vi "FGV_REWORK_DIAGNOSTICS_message_history_buffer.vi"(7 "options":T3, 8 "error_in":errorcluster, 11 "input":variant) -> (0 "error_out":errorcluster, 3 "message_history":T1[](array[typedef]))   [LabVIEW 2019]
uses:
  FGV_REWORK_DIAGNOSTICS_message_history_buffer.ctl
  REWORK_DIAGNOSTICS_message_history_buffer_all_info.ctl
  _misc/DIAGNOSTICS_message_type.ctl
  <userlib>/_OpenG.lib/array/array.llb/Filter 1D Array with Scalar (Variant)__ogtk.vi
  <vilib>/addons/database/_DB Variant To Data/Database Variant To Data.xnode
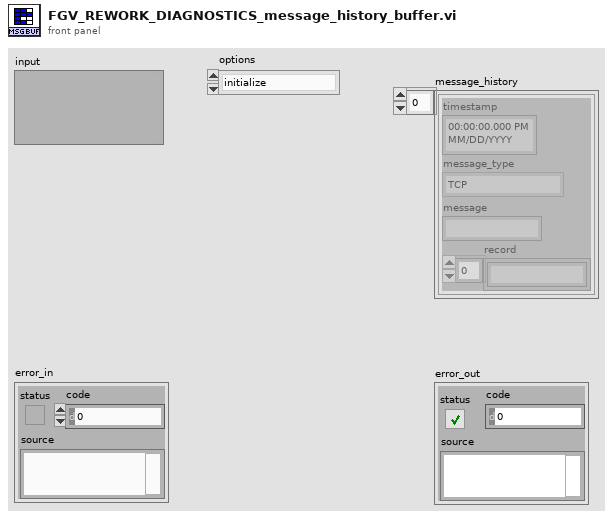
[diagram p1: front panel]
types:
  T1 = typedef "REWORK_DIAGNOSTICS_message_history_buffer_all_info.ctl" = cluster{"timestamp":timestamp, "message_type":T2, "message":string, "record":string[]}
  T2 = typedef "DIAGNOSTICS_message_type.ctl" = enum16{"TCP", "SQL"}
  T3 = typedef "FGV_REWORK_DIAGNOSTICS_message_history_buffer.ctl" = enum16{"initialize", "add_TCP_PLC_to_PC", "add_TCP_PC_to_PLC", "add_SQL_PC_to_DB", "add_SQL_transaction", "add_SQL_DB_to_PC", "get_all", "clear_all", "save_log"}
  T4 = enum16{"open", "replace", "create", "open or create", "replace or create", "replace or create with confirmation"}
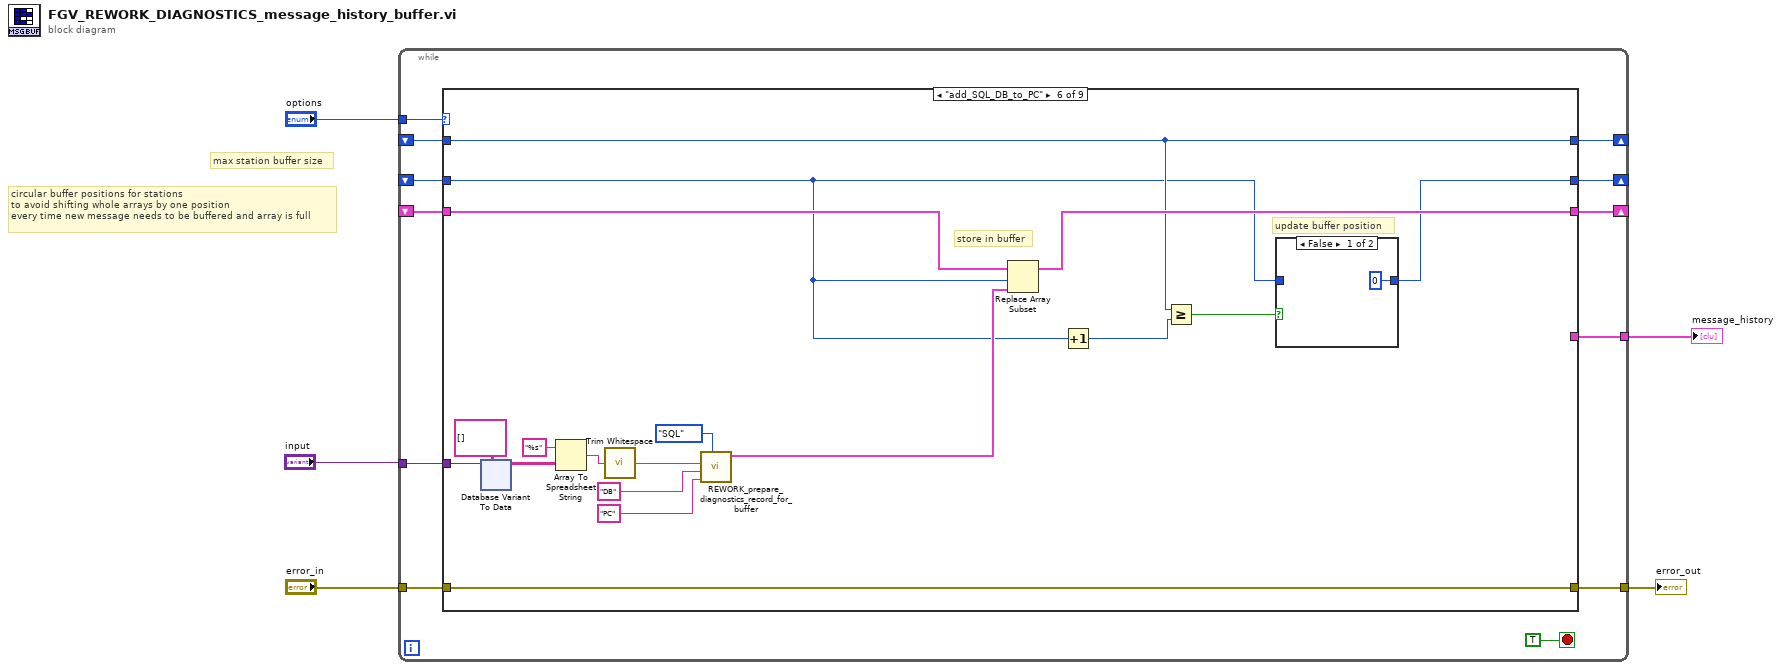
[diagram p0: block diagram]
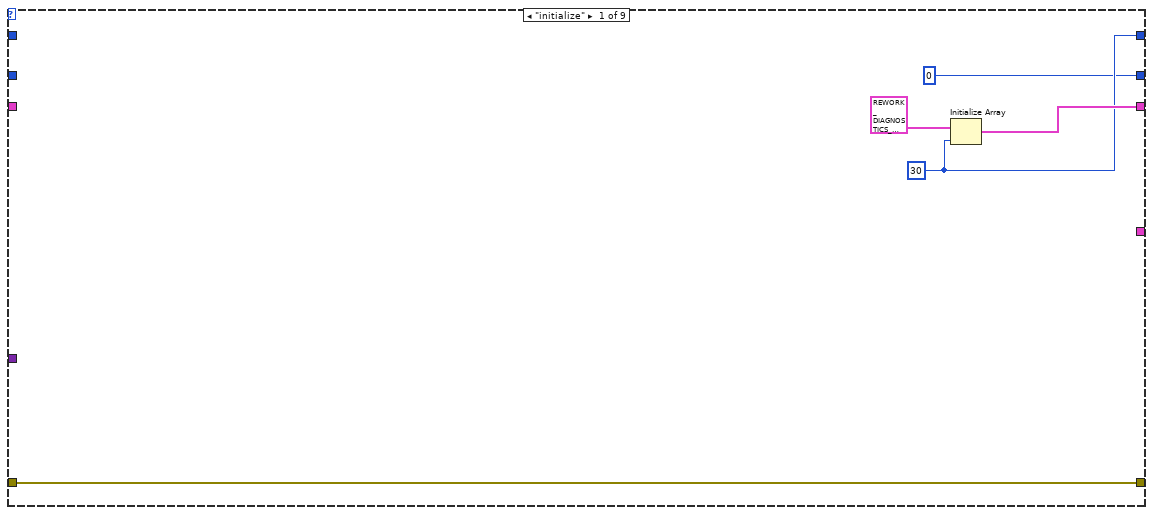
[diagram p2: hidden frame]
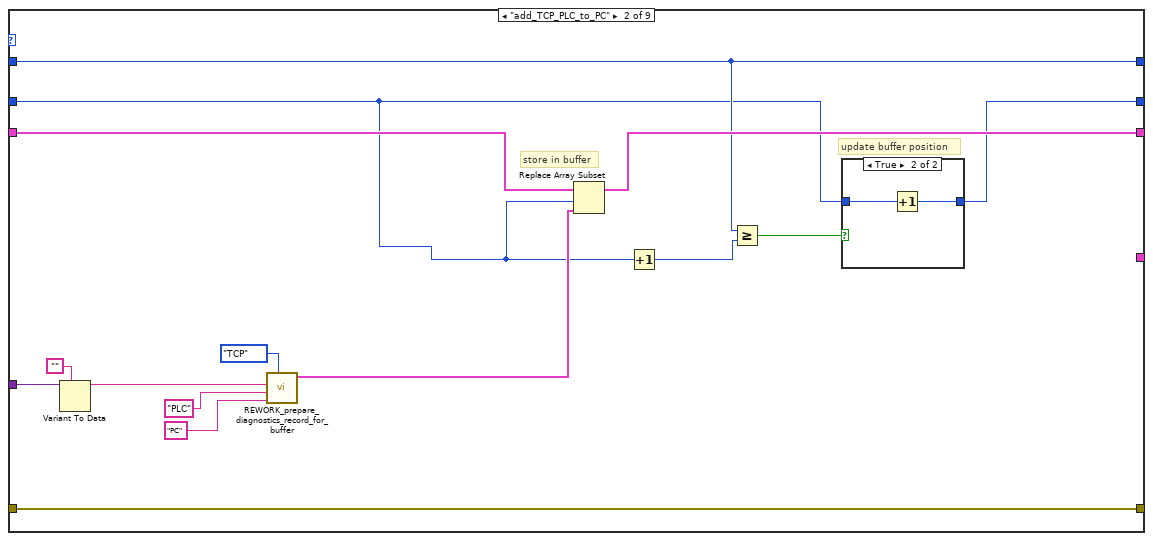
[diagram p3: hidden frame]
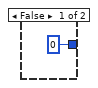
[diagram p4: hidden frame]
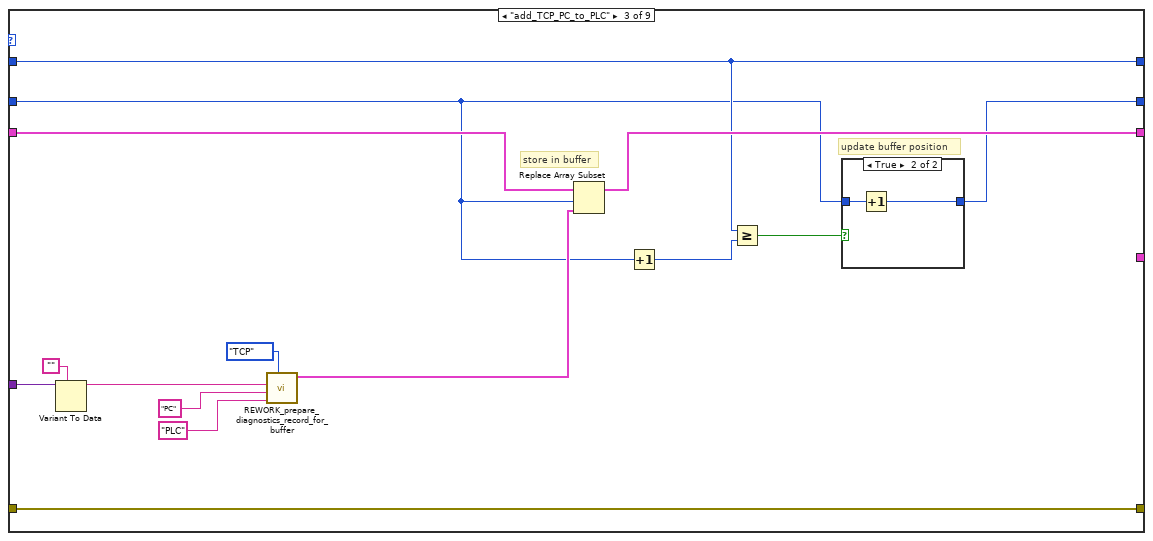
[diagram p5: hidden frame]
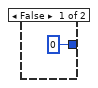
[diagram p6: hidden frame]
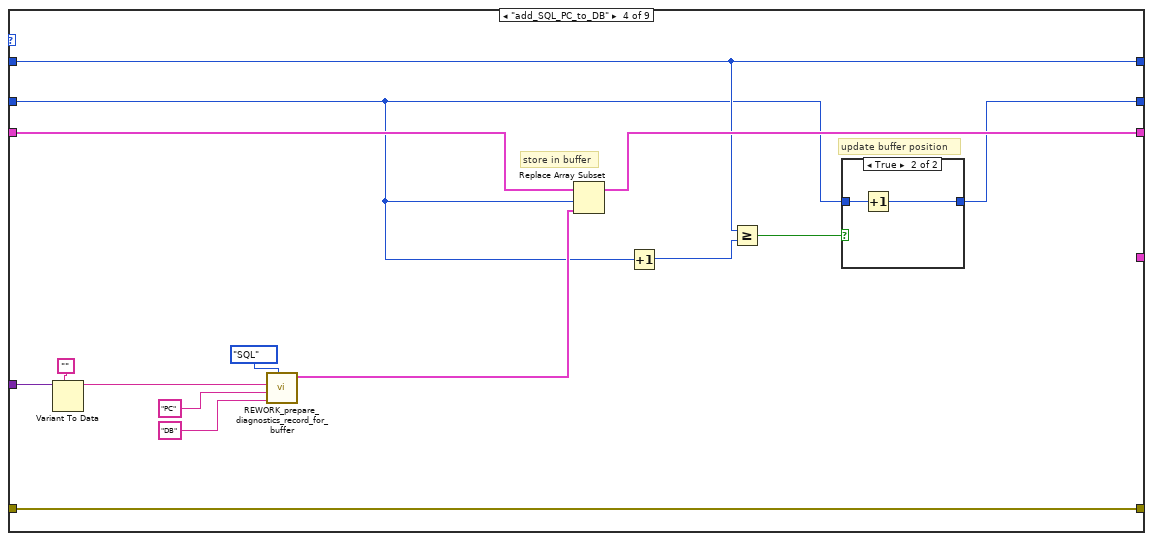
[diagram p7: hidden frame]
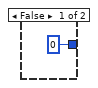
[diagram p8: hidden frame]
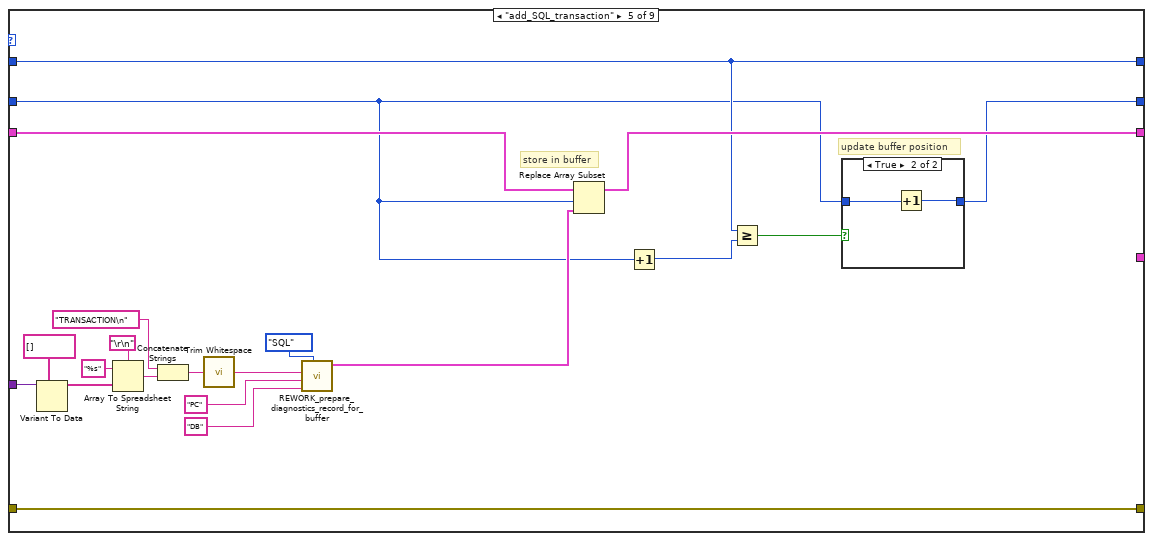
[diagram p9: hidden frame]
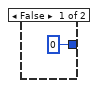
[diagram p10: hidden frame]
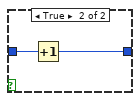
[diagram p11: hidden frame]
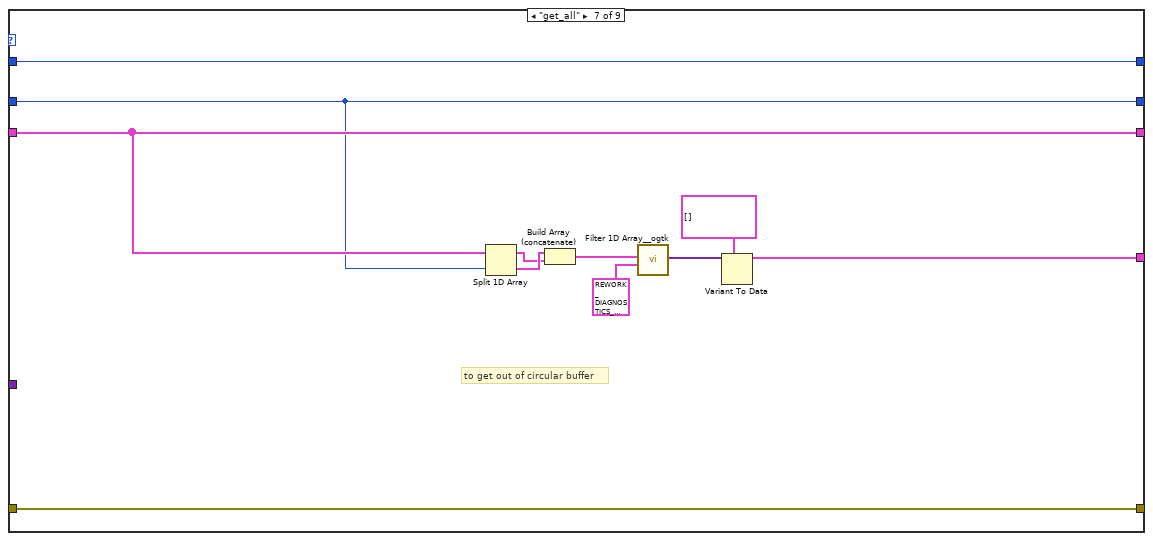
[diagram p12: hidden frame]
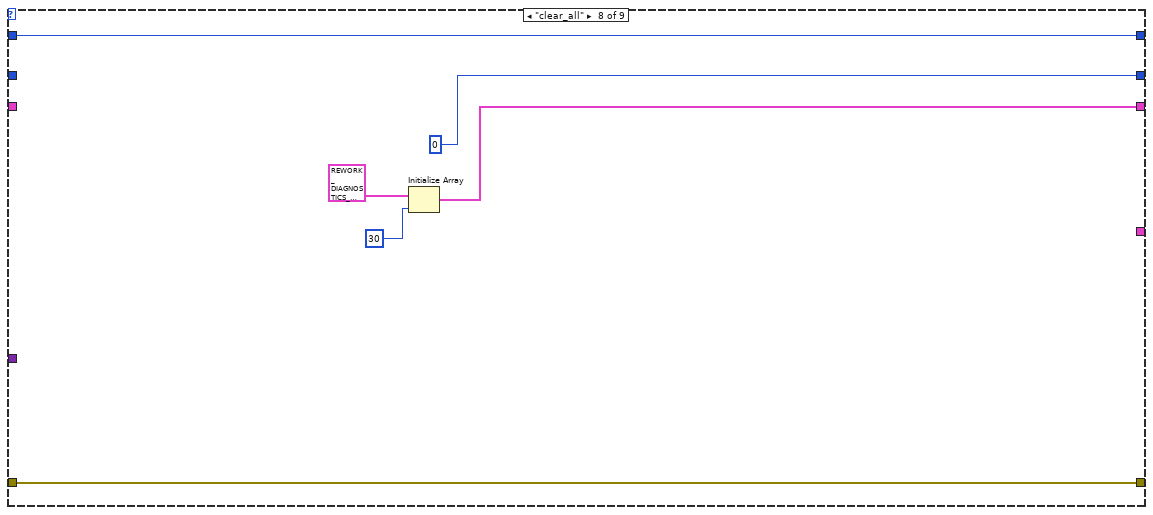
[diagram p13: hidden frame]
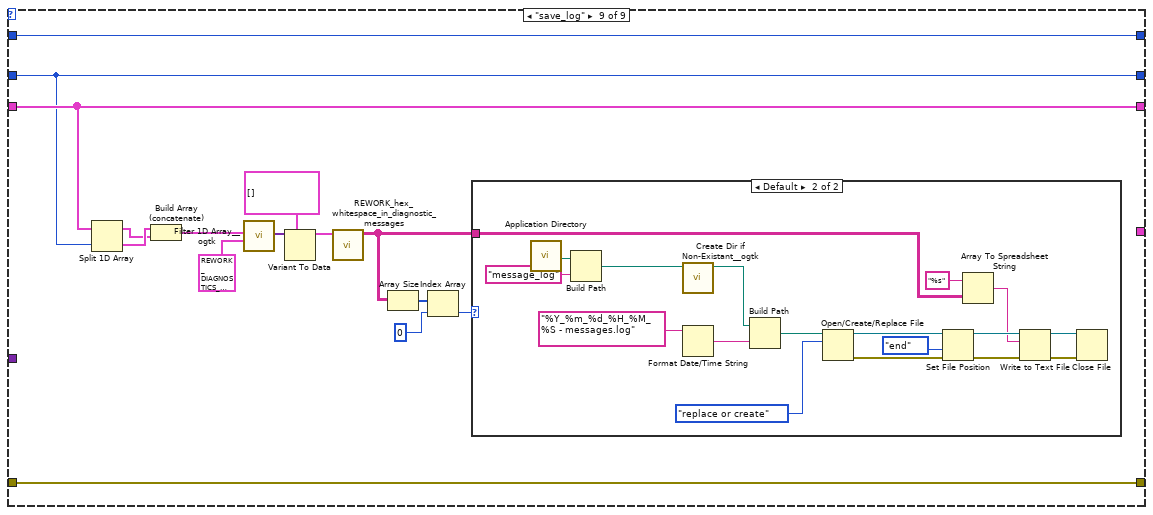
[diagram p14: hidden frame]
diagram:
  # "max station buffer size"
  # "circular buffer positions for stations\nto avoid shifting whole arrays by one position\nevery time new message needs to be buffered and array is full"
  n1 = while {
    tunnel: "options" -> [w16]
    tunnel: [w15] -> w5
    tunnel: "error_in" -> [w14]
    shift-right: [w13] -> _
    shift-left: _ -> [w12]
    tunnel: [w11] -> w2
    shift-right: [w10] -> _
    shift-left: _ -> [w9]
    tunnel: "input" -> [w8]
    shift-right: [w7] -> _
    shift-left: _ -> [w6]
    stop <- TRUE stop-if-true
    n2 = case shown="\"add_SQL_DB_to_PC\"" w16 {
      tunnel: [w22 w37 w55 w73 w97 w118 w164 w170 w185] -> w15
      tunnel: w14 -> [w22 w37 w55 w73 w97 w118 w164 w170 w185]
      tunnel: [w20 w33 w53 w71 w95 w116 w155 w165 w173] -> w13
      tunnel: w12 -> [_ w36 w54 w72 w96 w117 w155 _ w173]
      tunnel: [_ _ _ _ _ _ w156 _ _] -> w11
      tunnel: [0 w30 w52 w70 w94 w115 w154 0 w172] -> w10
      tunnel: w9 -> [_ w25 w43 w61 w79 w103 w154 _ w172]
      tunnel: w8 -> [_ w28 w45 w63 w88 w108 _ _ _]
      tunnel: [w19 w29 w51 w69 w93 w114 w163 w169 w184] -> w7
      tunnel: w6 -> [_ w29 w51 w69 w93 w114 w163 w169 w184]
      frame "initialize" {
        w19 = 30 ("dimension size")
        n3 = Initialize Array(T1 {"timestamp"=timestamp(0 s since 1904-01-01), "message_type"=enum."TCP", "message"="", "record"=[]} ("Cluster"), w19) -> (w20:T1[])
      }
      frame "add_TCP_PLC_to_PC" {
        # "update buffer position"
        # "store in buffer"
        n4 = Variant To Data(type="", Variant=w28) -> (data=w27:string)  [unwired: 1 in, 1 out]
        n5 = call "REWORK_prepare_diagnostics_record_for_buffer.vi"("message_type"=DIAGNOSTICS_message_type."TCP", "to"="PC" ("element"), "from"="PLC" ("element"), "message"=w27) -> ("record"=w35:T1)  [unwired: 7 in]
        n6 = Replace Array Subset(array=w36, new element=w35, index=w25) -> (w33:T1[])
        n7 = Increment(x=w25) -> (x+1=w32:i32)
        n8 = Greater Or Equal?(x=w29, y=w32) -> (x >= y?=w31:bool)
        n9 = case shown="True" w31 {
          tunnel: w25 -> [_ w40]
          tunnel: [0 ("array out") w39] -> w30
          frame False {
          }
          frame True {
            n10 = Increment(x=w40) -> (x+1=w39:i32)
          }
        }
      }
      frame "add_TCP_PC_to_PLC" {
        # "update buffer position"
        # "store in buffer"
        n11 = Variant To Data(type="", Variant=w45) -> (data=w44:string)  [unwired: 1 in, 1 out]
        n12 = call "REWORK_prepare_diagnostics_record_for_buffer.vi"("message_type"=DIAGNOSTICS_message_type."TCP", "to"="PLC" ("element"), "from"="PC" ("element"), "message"=w44) -> ("record"=w50:T1)  [unwired: 7 in]
        n13 = Replace Array Subset(array=w54, new element=w50, index=w43) -> (w53:T1[])
        n14 = Increment(x=w43) -> (x+1=w48:i32)
        n15 = Greater Or Equal?(x=w51, y=w48) -> (x >= y?=w47:bool)
        n16 = case shown="True" w47 {
          tunnel: w43 -> [_ w58]
          tunnel: [0 ("array out") w57] -> w52
          frame False {
          }
          frame True {
            n17 = Increment(x=w58) -> (x+1=w57:i32)
          }
        }
      }
      frame "add_SQL_PC_to_DB" {
        # "update buffer position"
        # "store in buffer"
        n18 = Variant To Data(type="", Variant=w63) -> (data=w62:string)  [unwired: 1 in, 1 out]
        n19 = call "REWORK_prepare_diagnostics_record_for_buffer.vi"("message_type"=DIAGNOSTICS_message_type."SQL", "to"="DB" ("element"), "from"="PC" ("element"), "message"=w62) -> ("record"=w68:T1)  [unwired: 7 in]
        n20 = Replace Array Subset(array=w72, new element=w68, index=w61) -> (w71:T1[])
        n21 = Increment(x=w61) -> (x+1=w66:i32)
        n22 = Greater Or Equal?(x=w69, y=w66) -> (x >= y?=w65:bool)
        n23 = case shown="True" w65 {
          tunnel: w61 -> [_ w76]
          tunnel: [0 ("array out") w75] -> w70
          frame False {
          }
          frame True {
            n24 = Increment(x=w76) -> (x+1=w75:i32)
          }
        }
      }
      frame "add_SQL_transaction" {
        # "update buffer position"
        # "store in buffer"
        n25 = Variant To Data(type=string[] [], Variant=w88) -> (data=w86:string[])  [unwired: 1 in, 1 out]
        n26 = Array To Spreadsheet String(delimiter (Tab)="\r\n", array=w86, 3:"%s" ("format string")) -> (spreadsheet string=w83:string)
        n27 = Concatenate Strings("TRANSACTION\n" ("string"), w83) -> (w81:string)
        n28 = call <vilib>:"Trim Whitespace.vi"("string"=w81) -> ("trimmed string"=w80:string)  [unwired: 1 in]
        n29 = call "REWORK_prepare_diagnostics_record_for_buffer.vi"("message_type"=DIAGNOSTICS_message_type."SQL", "to"="DB" ("element"), "from"="PC" ("element"), "message"=w80) -> ("record"=w92:T1)  [unwired: 7 in]
        n30 = Replace Array Subset(array=w96, new element=w92, index=w79) -> (w95:T1[])
        n31 = Increment(x=w79) -> (x+1=w90:i32)
        n32 = Greater Or Equal?(x=w93, y=w90) -> (x >= y?=w89:bool)
        n33 = case shown="True" w89 {
          tunnel: w79 -> [_ w100]
          tunnel: [0 ("array out") w99] -> w94
          frame False {
          }
          frame True {
            n34 = Increment(x=w100) -> (x+1=w99:i32)
          }
        }
      }
      frame "add_SQL_DB_to_PC" {
        # "update buffer position"
        # "store in buffer"
        n35 = xnode "Database Variant To Data"("database variant"=w108, "type"=string[][] []) -> ("data"=w107:string[][])  [unwired: 1 in, 1 out]
        n36 = Array To Spreadsheet String(array=w107, 3:"%s" ("format string")) -> (spreadsheet string=w104:string)  [unwired: 1 in]
        n37 = call <vilib>:"Trim Whitespace.vi"("string"=w104) -> ("trimmed string"=w105:string)  [unwired: 1 in]
        n38 = call "REWORK_prepare_diagnostics_record_for_buffer.vi"("message_type"=DIAGNOSTICS_message_type."SQL", "to"="PC" ("element"), "from"="DB" ("element"), "message"=w105) -> ("record"=w113:T1)  [unwired: 7 in]
        n39 = Replace Array Subset(array=w117, new element=w113, index=w103) -> (w116:T1[])
        n40 = Increment(x=w103) -> (x+1=w111:i32)
        n41 = Greater Or Equal?(x=w114, y=w111) -> (x >= y?=w110:bool)
        n42 = case shown="False" w110 {
          tunnel: w103 -> [_ w153]
          tunnel: [0 ("array out") w152] -> w115
          frame False {
          }
          frame True {
            n43 = Increment(x=w153) -> (x+1=w152:i32)
          }
        }
      }
      frame "get_all" {
        # "to get out of circular buffer"
        n44 = Split 1D Array(array=w155, index=w154) -> (first subarray=w161:T1[], second subarray=w162:T1[])
        n45 = Build Array (concatenate)(w162, w161) -> (w160:T1[])
        n46 = call-poly <userlib>:"Filter 1D Array__ogtk.vi"("items to filter"=T1 {"timestamp"=timestamp(0 s since 1904-01-01), "message_type"=enum."TCP", "message"="", "record"=[]} ("Cluster"), "array"=w160) -> ("filtered array"=w158:variant[])  [unwired: 4 in, 1 out]
        n47 = Variant To Data(type=T1[] [], Variant=w158) -> (data=w156:T1[])  [unwired: 1 in, 1 out]
      }
      frame "clear_all" {
        n48 = Initialize Array(T1 {"timestamp"=timestamp(0 s since 1904-01-01), "message_type"=enum."TCP", "message"="", "record"=[]} ("Cluster"), 30 ("dimension size")) -> (w165:T1[])
      }
      frame "save_log" {
        n49 = Split 1D Array(array=w173, index=w172) -> (first subarray=w178:T1[], second subarray=w179:T1[])
        n50 = Build Array (concatenate)(w179, w178) -> (w177:T1[])
        n51 = call-poly <userlib>:"Filter 1D Array__ogtk.vi"("items to filter"=T1 {"timestamp"=timestamp(0 s since 1904-01-01), "message_type"=enum."TCP", "message"="", "record"=[]} ("Cluster"), "array"=w177) -> ("filtered array"=w175:variant[])  [unwired: 4 in, 1 out]
        n52 = Variant To Data(type=T1[] [], Variant=w175) -> (data=w171:T1[])  [unwired: 1 in, 1 out]
        n53 = call "REWORK_hex_whitespace_in_diagnostic_messages.vi"("message_history"=w171) -> ("hexed_records"=w180:string[][])  [unwired: 10 in]
        n54 = Array Size(array=w180) -> (size(s)=w183:i32[])
        n55 = Index Array(array=w183, index=0) -> (element=w181:i32)
        n56 = case shown="Default" w181 {
          tunnel: w180 -> [_ w203]
          frame 0 {
          }
          frame Default {
            n57 = call <vilib>:"Application Directory.vi"() -> ("Application Directory"=w189:path)
            n58 = Build Path(base path=w189, name or relative path="message_log") -> (appended path=w187:path)
            n59 = call <userlib>:"Create Dir if Non-Existant__ogtk.vi"("Directory Path"=w187) -> ("dup Directory Path"=w186:path)  [unwired: 8 in, 2 out]
            n60 = Format Date/Time String(time format string (%c)="%Y_%m_%d_%H_%M_%S - messages.log") -> (date/time string=w190:string)  [unwired: 2 in]
            n61 = Build Path(base path=w186, name or relative path=w190) -> (appended path=w195:path)
            n62 = Open/Create/Replace File(file path (use dialog)=w195, operation (0:open)=T4."replace or create") -> (refnum out=w199:refnum<file>, error out=w196:errorcluster)  [unwired: 4 in, 1 out]
            n63 = Set File Position(refnum=w199, from (0:start)=enum16{"start", "end", "current"}."end", error in=w196) -> (refnum out=w201:refnum<file>, error out=w197:errorcluster)  [unwired: 1 in]
            n64 = Array To Spreadsheet String(array=w203, 3:"%s" ("format string")) -> (spreadsheet string=w192:string)  [unwired: 1 in]
            n65 = Write to Text File(file (use dialog)=w201, text=w192, error in=w197) -> (refnum out=w194:refnum<file>, error out=w193:errorcluster)  [unwired: 1 in, 1 out]
            n66 = Close File(refnum=w194, error in=w193) -> ()  [unwired: 2 out]
          }
        }
      }
    }
  }
  "error_out" <- w5
  "message_history" <- w2
